vi "Destroy User Events.vi"(11 "UI Template in":refnum<class "Object Dictionary UI.lvclass">) -> (3 "UI Template out":refnum<class "Object Dictionary UI.lvclass">)   [LabVIEW 2024, in "Object Dictionary UI.lvlib" / "Object Dictionary UI.lvclass"]
uses:
  Object Dictionary UI.lvclass
  Object Dictionary UI.lvclass/Object Dictionary UI.ctl
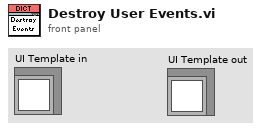
[diagram p1: front panel]
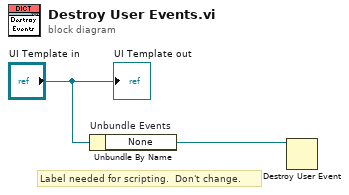
[diagram p0: block diagram]
diagram:
  # "Label needed for scripting.  Don't change."
  n1 = Unbundle By Name "Unbundle Events"("UI Template in") -> ("None"=w2:refnum<user-event>)
  n2 = Destroy User Event(user event=w2) -> ()  [unwired: 1 in, 1 out]
  "UI Template out" <- "UI Template in"
